vi "List Threads.vi"() -> ()   [LabVIEW 2018]
doc: "©2019\nWiebe Walstra\nwww.carya.nl"
uses:
  LogonUser.lvclass
  Threads.ctl
panel:
  out "Ticks":i64[](array[numeric])
  out "IDs":i32[](array[numeric])
  out "list files":errorcluster[](array[cluster])
  out "read files":errorcluster[](array[cluster])
  out "Array 3":i64[](array[numeric])
  out "Count":i32
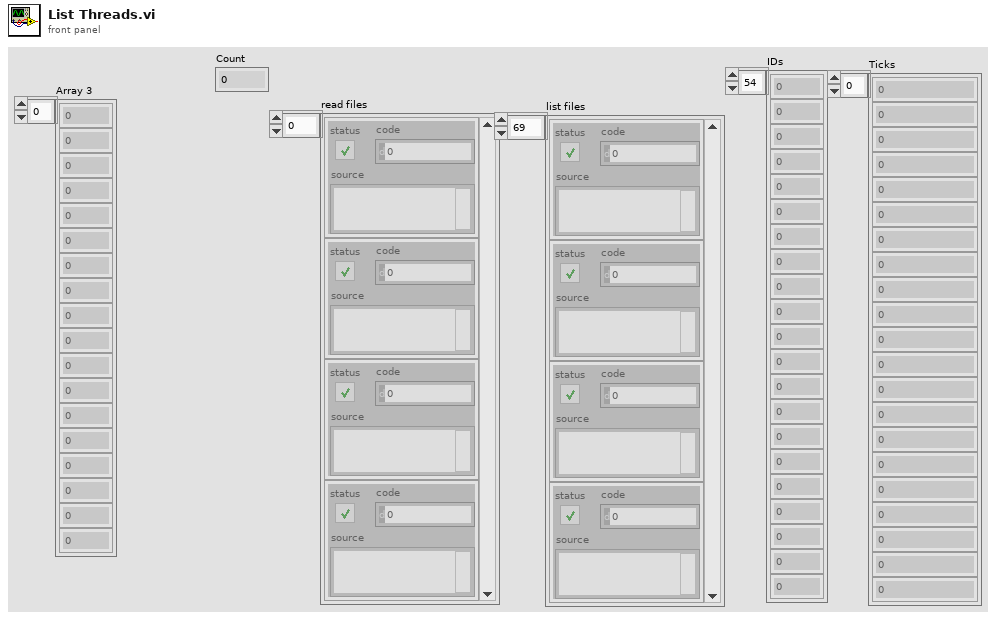
[diagram p1: front panel]
types:
  T1 = enum32{"user interface", "standard", "instrument i/o", "data acquisition", "other 1", "other 2", "same as caller"}
  T2 = typedef "LogonUser.lvclass/Threads.ctl" = enum32{"user interface", "standard", "instrument i/o", "data acquisition", "other 1", "other 2", "same as caller", "manual"}
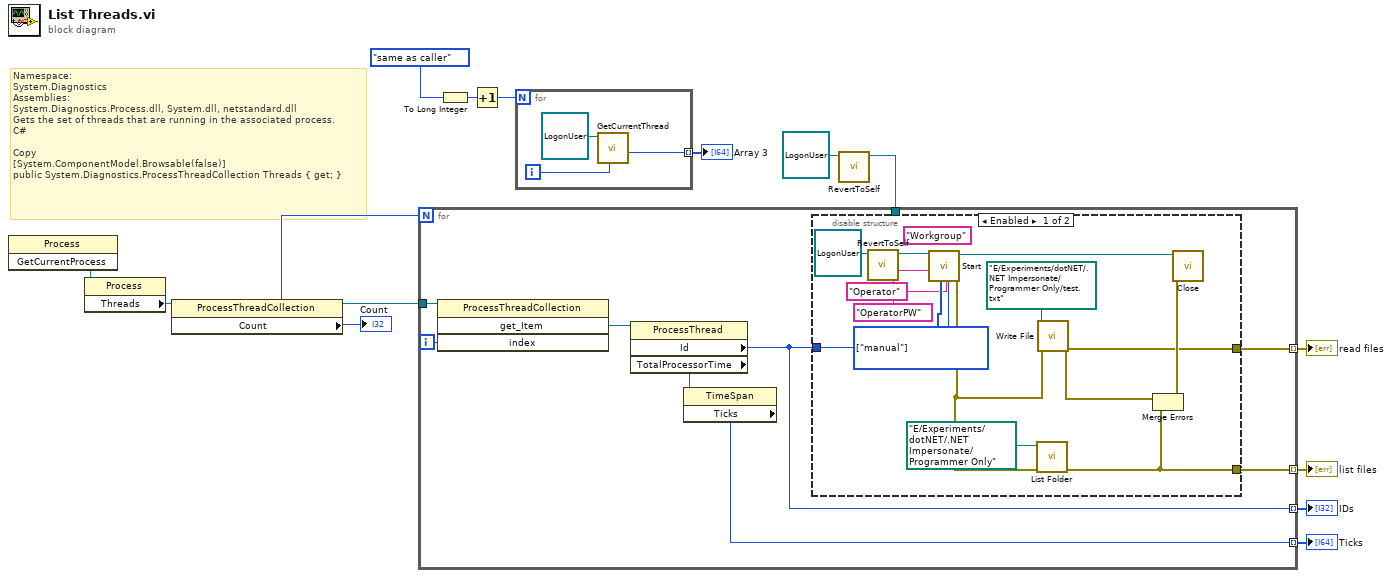
[diagram p0: block diagram]
diagram:
  # "Namespace:\nSystem.Diagnostics \nAssemblies:\nSystem.Diagnostics.Process.dll, System.dll, netstandard.dll\nGets the set of threads that are running in the associated process.\nC#\n\nCopy\n[System.ComponentModel.Browsable(false)]\npublic System.Diagnostics.ProcessThreadCollection Threads { get; }"
  n1 = invoke class="Process" method="GetCurrentProcess"() -> ("GetCurrentProcess"=w14:refnum<k24>)  [unwired: 3 in, 2 out]
  n2 = property class="Process"(reference=w14) -> ("Threads"=w6:refnum<k24>)  [unwired: 1 in, 2 out]
  n3 = property class="ProcessThreadCollection"(reference=w6) -> (reference out=w13:refnum<k24>, "Count"=w12:i32)  [unwired: 1 in, 1 out]
  "Count" <- w12
  n4 = To Long Integer(number=T1."same as caller" ("Thread")) -> (32bit integer=w5:i32)
  n5 = Increment(x=w5) -> (x+1=w4:i32)
  n6 = for {
    N: w4 -> [_]
    tunnel: [w15] -> w3 mode=indexing
    i -> [w16]
    n7 = call-dynamic "GetCurrentThread.vi"("Thread"=w16, "Impersonate in"=refnum<class "LogonUser.lvclass"> refnum) -> ("thread id"=w15:i64)  [unwired: 7 in, 2 out]
  }
  "Array 3" <- w3
  n8 = call-dynamic "RevertToSelf.vi"("Impersonate in"=refnum<class "LogonUser.lvclass"> refnum) -> ("Impersonate out"=w2:refnum<class "LogonUser.lvclass">)  [unwired: 9 in, 1 out]
  n9 = for {
    N: w12 -> [_]
    tunnel: w13 -> [w25]
    tunnel: [w21] -> w10 mode=indexing
    tunnel: [w20] -> w9 mode=indexing
    tunnel: [w19] -> w8 mode=indexing
    tunnel: [w18] -> w7 mode=indexing
    tunnel: w2 -> [_]
    i -> [w24]
    n10 = invoke class="ProcessThreadCollection" method="get_Item"(reference=w25, "index"=w24) -> ("get_Item"=w23:refnum<k24>)  [unwired: 2 in, 3 out]
    n11 = property class="ProcessThread"(reference=w23) -> ("Id"=w19:i32, "TotalProcessorTime"=w22:refnum<k24>)  [unwired: 1 in, 2 out]
    n12 = property class="TimeSpan"(reference=w22) -> ("Ticks"=w18:i64)  [unwired: 1 in, 2 out]
    n13 = disable-structure shown="Enabled" {
      disable-tunnel: [w29 _] -> w21
      disable-tunnel: [w28 _] -> w20
      disable-tunnel: w19 -> [w26 _]
      frame Enabled {
        (unwired) "Workgroup" ("domainName")
        w35 = T2[] [enum."manual"] items=["user interface", "standard", "instrument i/o", "data acquisition", "other 1", "other 2", "same as caller", "manual"] ("Thread")
        n14 = call-dynamic "RevertToSelf.vi"("Impersonate in"=refnum<class "LogonUser.lvclass"> refnum) -> ("Impersonate out"=w27:refnum<class "LogonUser.lvclass">)  [unwired: 9 in, 1 out]
        n15 = call-dynamic "Start.vi"("Manual thread"=w26, "Thread"=w35, "password"="OperatorPW", "userName"="Operator", "Impersonate in"=w27) -> ("error out"=w38:errorcluster, "Impersonate out"=w36:refnum<class "LogonUser.lvclass">)  [unwired: 5 in]
        n16 = call "List Folder.vi"("error in (no error)"=w38, "path"=path "E:/Experiments/dotNET/.NET Impersonate/Programmer Only") -> ("error out"=w28:errorcluster)  [unwired: 9 in]
        n17 = call "Write File.vi"("error in (no error)"=w38, "path"=path "E:/Experiments/dotNET/.NET Impersonate/Programmer Only/test.txt") -> ("error out"=w29:errorcluster)  [unwired: 9 in]
        n18 = Merge Errors(w29, w28) -> (w37:errorcluster)
        n19 = call-dynamic "Close.vi"("error in (no error)"=w37, "Impersonate in"=w36) -> ()  [unwired: 8 in, 2 out]
      }
      frame Disabled {
      }
    }
  }
  "read files" <- w10
  "list files" <- w9
  "IDs" <- w8
  "Ticks" <- w7
